vi "App_Snap.vi"(8 "error in":errorcluster, 11 "Image":T1) -> (0 "error out":errorcluster)   [LabVIEW 2015, in "Application 1.lvlib"]
uses:
  Application 1.lvlib
  <vilib>/vision/Image Controls.llb/IMAQ Image.ctl
  <vilib>/userdefined/High Color/IMAQdx.ctl
  <vilib>/vision/driver/IMAQdx.llb/IMAQdx Acquisition Mode.ctl
  <vilib>/vision/driver/IMAQdx.llb/IMAQdx Buffer Number Mode.ctl
  <vilib>/vision/driver/NI_Vision_Acquisition_Software.lvlib
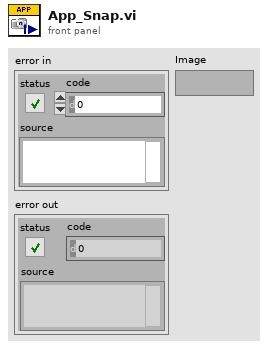
[diagram p1: front panel]
types:
  T1 = typedef "IMAQ Image.ctl" = refnum<image>
  T2 = cluster{"Type":u32, "Version":u32, "Flags":u32, "SerialNumberHigh":u32, "SerialNumberLow":u32, "BusType":u32, "InterfaceName":string, "VendorName":string, "ModelName":string, "CameraFileName":string, "CameraAttributeURL":string}[]
  T3 = typedef "NI_Vision_Acquisition_Software.lvlib/IMAQdx Buffer Number Mode.ctl" = enum32{"Next", "Last", "Buffer Number", "Every", "Last New"}
  T4 = typedef "NI_Vision_Acquisition_Software.lvlib/IMAQdx Acquisition Mode.ctl" = enum32{"One Shot", "Continuous"}
  T5 = typedef "IMAQdx.ctl" = refnum<k21>
  T6 = cluster{"Type":u32, "Version":u32, "Flags":u32, "SerialNumberHigh":u32, "SerialNumberLow":u32, "BusType":u32, "InterfaceName":string, "VendorName":string, "ModelName":string, "CameraFileName":string, "CameraAttributeURL":string}
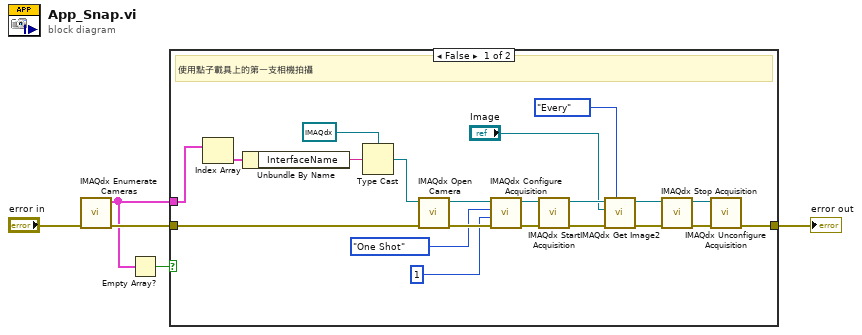
[diagram p0: block diagram]
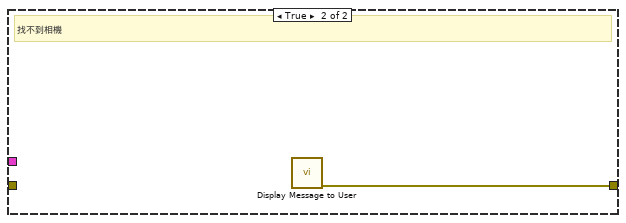
[diagram p2: hidden frame]
diagram:
  n1 = call <vilib>:"IMAQdx Enumerate Cameras.vi"("error in"="error in") -> ("error out"=w3:errorcluster, "Camera Information Array"=w2:T2)  [unwired: 9 in]
  n2 = Empty Array?(array=w2) -> (empty?=w4:bool)
  n3 = case shown="False" w4 {
    tunnel: w3 -> [w22 _]
    tunnel: w2 -> [w26 _]
    tunnel: [w6 w27] -> w1
    frame False {
      # "使用點子載具上的第一支相機拍攝"
      n4 = Index Array(array=w26) -> (element=w25:T6)  [unwired: 1 in]
      n5 = Unbundle By Name(w25) -> ("InterfaceName"=w24:string)
      n6 = Type Cast(type=T5 refnum ("Session In"), x=w24) -> (*(type *) &x=w21:T5)
      n7 = call <vilib>:"IMAQdx Open Camera.vi"("error in"=w22, "Session In"=w21) -> ("error out"=w12:errorcluster, "Session Out"=w11:T5)  [unwired: 8 in]
      n8 = call <vilib>:"IMAQdx Configure Acquisition.vi"("error in"=w12, "Number of Buffers"=u32 1, "Continuous?"=IMAQdx_Acquisition_Mode."One Shot", "Session In"=w11) -> ("error out"=w19:errorcluster, "Session Out"=w20:T5)  [unwired: 6 in]
      n9 = call <vilib>:"IMAQdx Start Acquisition.vi"("error in"=w19, "Session In"=w20) -> ("error out"=w17:errorcluster, "Session Out"=w18:T5)  [unwired: 8 in]
      n10 = call <vilib>:"IMAQdx Get Image2.vi"("Buffer Number Mode (Next)"=IMAQdx_Buffer_Number_Mode."Every", "error in"=w17, "Image In"="Image", "Session In"=w18) -> ("error out"=w15:errorcluster, "Session Out"=w16:T5)  [unwired: 4 in, 2 out]
      n11 = call <vilib>:"IMAQdx Stop Acquisition.vi"("error in"=w15, "Session In"=w16) -> ("error out"=w13:errorcluster, "Session Out"=w14:T5)  [unwired: 8 in]
      n12 = call <vilib>:"IMAQdx Unconfigure Acquisition.vi"("error in"=w13, "Session In"=w14) -> ("error out"=w6:errorcluster)  [unwired: 8 in, 1 out]
    }
    frame True {
      # "找不到相機"
      n13 = call "Display Message to User"() -> ("error out"=w27:errorcluster)  [unwired: 10 in, 1 out]
    }
  }
  "error out" <- w1
